vi "CheckPossibleBalls.vi"(1 "max ball vel":dbl, 8 "Fps":dbl=40.0, 9 "Field Size":T3, 10 "Array of cameras":T4[](array[typedef]) {"robots_blue"."height" format="%+4.3f"; "robots_blue"."pixel_y" format="%+4.3f"; "robots_blue"."pixel_x" format="%+4.3f"; "robots_blue"."orientation" format="%+4.3f"; "robots_blue"."y" format="%+4.3f"; "robots_blue"."confidence" format="%4.3f"; "robots_blue"."x" format="%+4.3f"; "robots_yellow"."height" format="%+4.3f"; "robots_yellow"."pixel_y" format="%+4.3f"; "robots_yellow"."pixel_x" format="%+4.3f"; "robots_yellow"."orientation" format="%+4.3f"; "robots_yellow"."y" format="%+4.3f"; "robots_yellow"."confidence" format="%4.3f"; "robots_yellow"."x" format="%+4.3f"}, 11 "last ball choosed by mediacameras":T1[](array[typedef])) -> (2 "sum":i32, 3 "Detection Frame In out":T4[](array[typedef]) {"robots_blue"."height" format="%+4.3f"; "robots_blue"."pixel_y" format="%+4.3f"; "robots_blue"."pixel_x" format="%+4.3f"; "robots_blue"."orientation" format="%+4.3f"; "robots_blue"."y" format="%+4.3f"; "robots_blue"."confidence" format="%4.3f"; "robots_blue"."x" format="%+4.3f"; "robots_yellow"."height" format="%+4.3f"; "robots_yellow"."pixel_y" format="%+4.3f"; "robots_yellow"."pixel_x" format="%+4.3f"; "robots_yellow"."orientation" format="%+4.3f"; "robots_yellow"."y" format="%+4.3f"; "robots_yellow"."confidence" format="%4.3f"; "robots_yellow"."x" format="%+4.3f"})   [LabVIEW 2023]
uses:
  Vision_class/Old vision/Controls/SSL Detection Frame.ctl
  Vision_class/Old vision/Controls/SSL Detection Robot.ctl
  <vilib>/Analysis/Matrix/Datatypes/RealMatrix.ctl
  Vision_class/Old vision/Controls/SSL Detection Ball.ctl
  Utilities_class/Utilities.lvclass
  <vilib>/Analysis/Matrix/NI_Matrix.lvlib
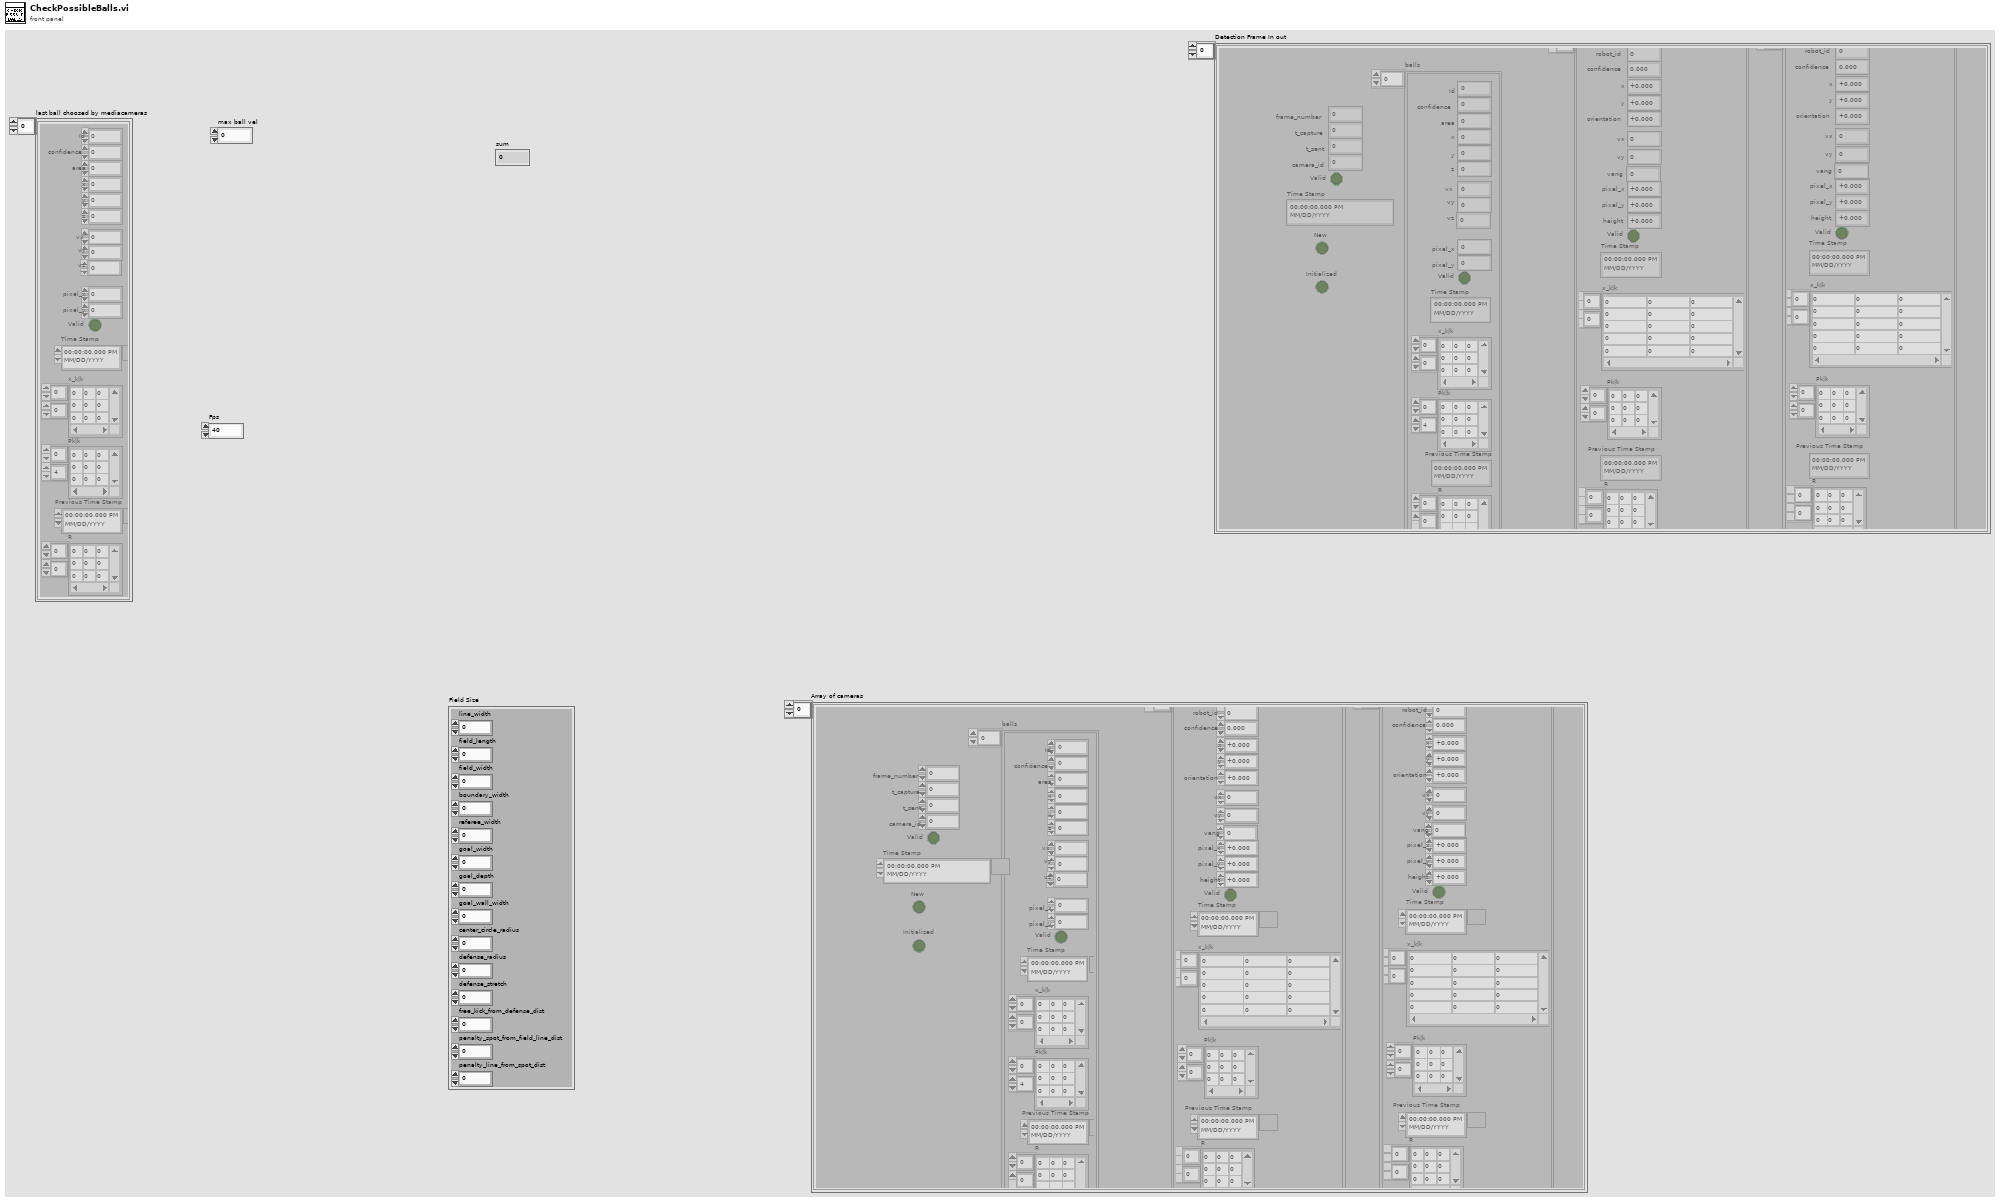
[diagram p1: front panel]
types:
  T1 = typedef "SSL Detection Ball.ctl" = cluster{"x":sgl, "area":u32, "confidence":sgl, "y":sgl, "z":sgl, "pixel_x":sgl, "pixel_y":sgl, "Valid":bool, "Time Stamp":timestamp, "x_k|k":T2, "Pk|k":T2, "Id":u32, "Previous Time Stamp":timestamp, "R":T2, " vx":sgl, "vy":dbl, "vz":dbl}
  T2 = typedef "NI_Matrix.lvlib/RealMatrix.ctl" = dbl[][]
  T3 = cluster{"line_width":u32, "field_length":u32, "field_width":u32, "boundary_width":u32, "referee_width":u32, "goal_width":u32, "goal_depth":u32, "goal_wall_width":u32, "center_circle_radius":u32, "defense_radius":u32, "defense_stretch":u32, "free_kick_from_defense_dist":u32, "penalty_spot_from_field_line_dist":u32, "penalty_line_from_spot_dist":u32}
  T4 = typedef "SSL Detection Frame.ctl" = cluster{"frame_number":u32, "t_capture":dbl, "t_sent":dbl, "camera_id":u32, "robots_yellow":T5[], "robots_blue":T5[], "balls":T1[], "Valid":bool, "Time Stamp":timestamp, "New":bool, "Initialized":bool}
  T5 = typedef "SSL Detection Robot.ctl" = cluster{"x":sgl, "robot_id":u32, "confidence":sgl, "y":sgl, "orientation":sgl, "pixel_x":sgl, "pixel_y":sgl, "height":sgl, "Valid":bool, "Time Stamp":timestamp, "x_k|k":T2, "Pk|k":T2, "Previous Time Stamp":timestamp, "R":T2, "vx":dbl, "vy":dbl, "vang":dbl}
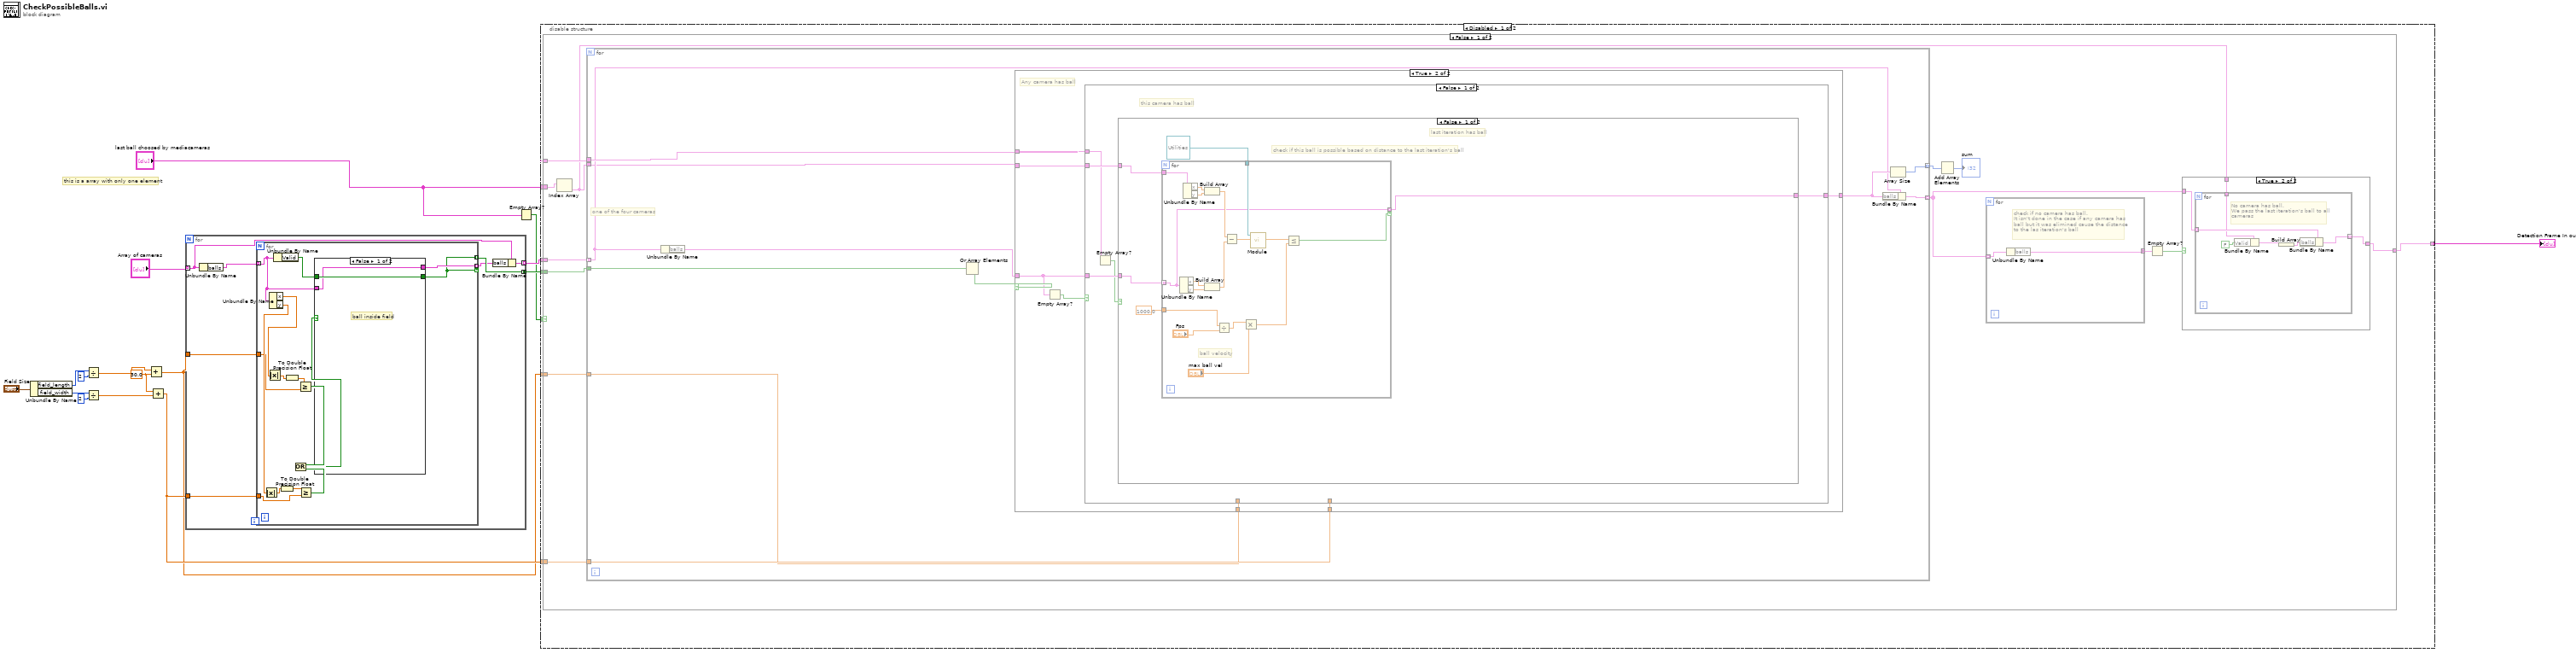
[diagram p0: block diagram]
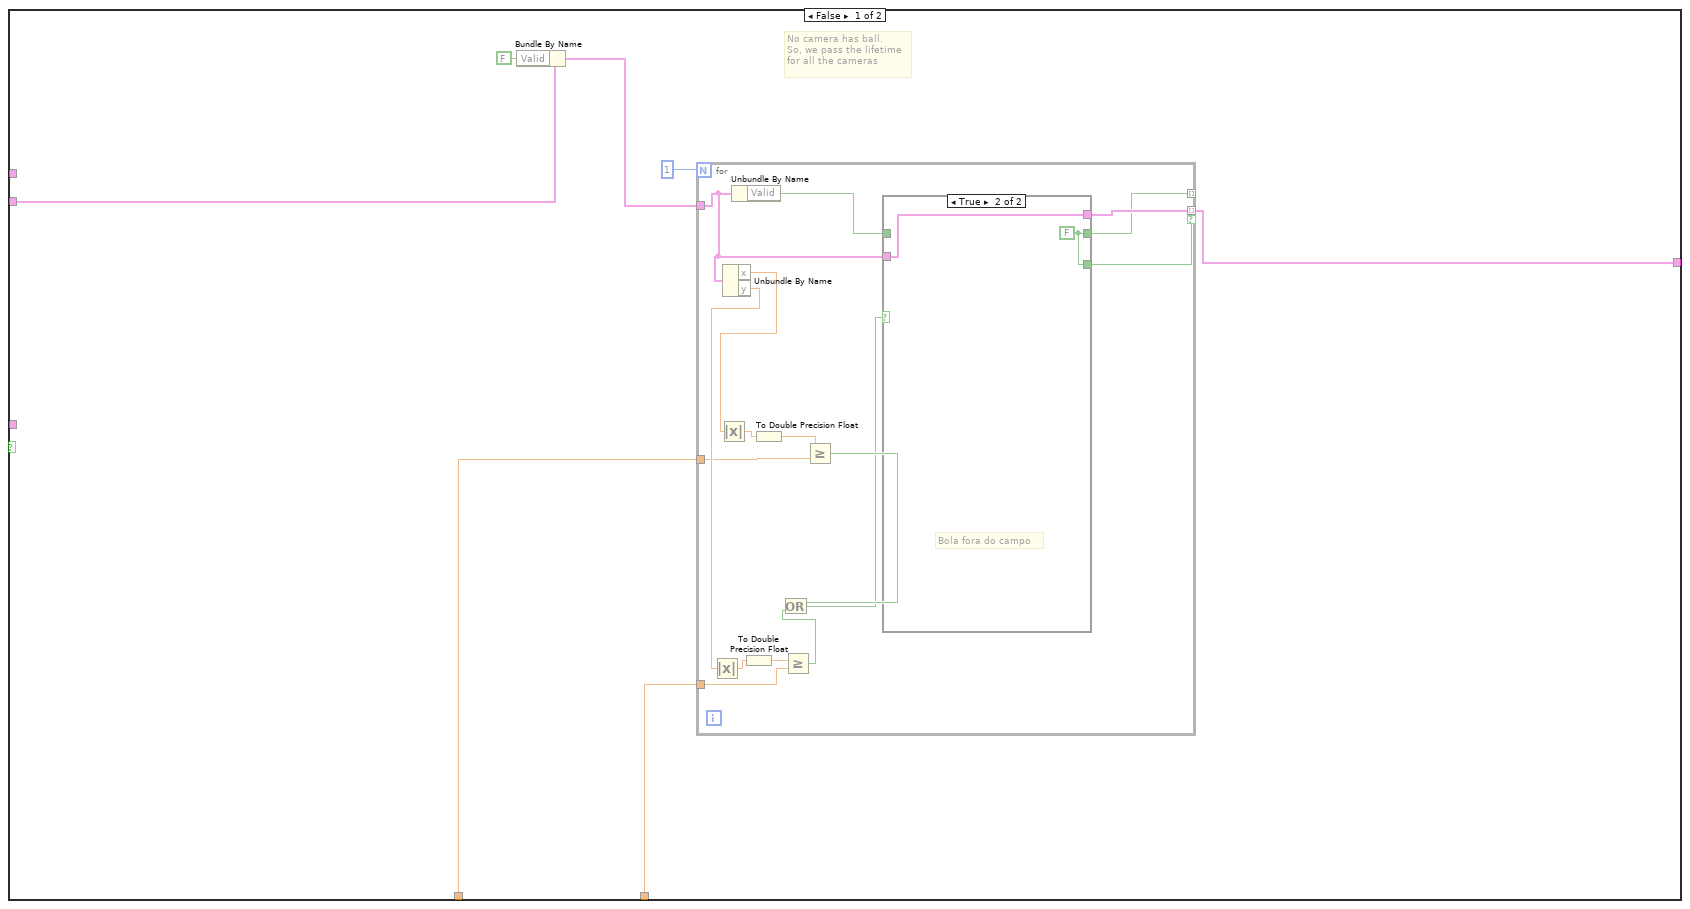
[diagram p3: hidden frame]
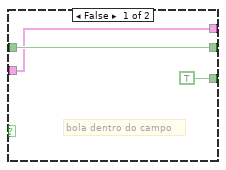
[diagram p4: hidden frame]
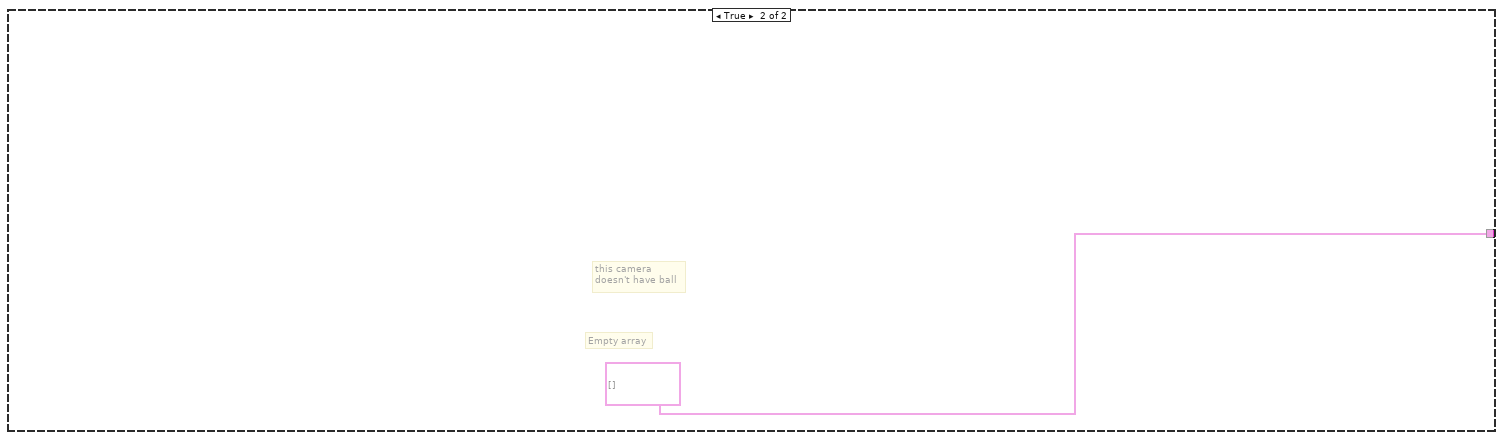
[diagram p6: hidden frame]
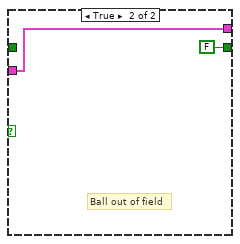
[diagram p9: hidden frame]
diagram:
  w10 = 30.0 ("y")
  # "this is a array with only one element"
  n1 = Unbundle By Name("Field Size") -> ("field_length"=w15:u32, "field_width"=w14:u32)
  n2 = Divide(x=w15, y=2) -> (x/y=w9:dbl)
  n3 = Divide(x=w14, y=2) -> (x/y=w11:dbl)
  n4 = Add(x=w9, y=w10) -> (x+y=w7:dbl)
  n5 = Add(x=w10, y=w11) -> (x+y=w8:dbl)
  n6 = for {
    tunnel: w8 -> [w23]
    tunnel: w7 -> [w22]
    tunnel: "Array of cameras" -> [w18] mode=indexing
    tunnel: [w17] -> w4 mode=indexing
    tunnel: [w20] -> w6 mode=concatenating
    n7 = Unbundle By Name(w18) -> ("balls"=w21:T1[])
    n8 = for {
      tunnel: w21 -> [w29] mode=indexing
      tunnel: [w26] -> w20 mode=indexing
      tunnel: [w37] -> w19 mode=indexing if=w26
      tunnel: w23 -> [w25]
      tunnel: w22 -> [w24]
      n9 = Unbundle By Name(w29) -> ("x"=w28:sgl, "y"=w27:sgl)
      n10 = Absolute Value(x=w27) -> (abs(x)=w33:sgl)
      n11 = Absolute Value(x=w28) -> (abs(x)=w32:sgl)
      n12 = Unbundle By Name(w29) -> ("Valid"=w38:bool)
      n13 = To Double Precision Float(number=w33) -> (double precision float=w34:dbl)
      n14 = To Double Precision Float(number=w32) -> (double precision float=w31:dbl)
      n15 = Greater Or Equal?(x=w31, y=w24) -> (x >= y?=w36:bool)
      n16 = Greater Or Equal?(x=w34, y=w25) -> (x >= y?=w35:bool)
      n17 = Or(x=w36, y=w35) -> (x .or. y?=w30:bool)
      n18 = case shown="False" w30 {
        tunnel: w38 -> [w40 _]
        tunnel: [w40 FALSE ("Valid")] -> w26
        tunnel: w29 -> [w39 w41]
        tunnel: [w39 w41] -> w37
        frame False {
          # "ball inside field"
        }
        frame True {
          # "Ball out of field"
        }
      }
    }
    n19 = Bundle By Name(cluster=w18, "balls"=w19) -> (w17:T4)
  }
  n20 = Empty Array?(array="last ball choosed by mediacameras") -> (empty?=w3:bool)
  n21 = disable-structure shown="Disabled" {
    disable-tunnel: w8 -> [w49 _]
    disable-tunnel: w7 -> [w48 _]
    disable-tunnel: w6 -> [w47 _]
    disable-tunnel: w4 -> [w46 w151]
    disable-tunnel: w3 -> [w45 _]
    disable-tunnel: "last ball choosed by mediacameras" -> [w44 _]
    disable-tunnel: [w43 w151] -> w1
    frame Disabled {
      n22 = case shown="False" w45 {
        tunnel: w49 -> [w60 _]
        tunnel: w48 -> [w59 _]
        tunnel: w47 -> [w58 _]
        tunnel: w44 -> [w54 _]
        tunnel: [w53 w150] -> w43
        tunnel: w46 -> [w52 w150]
        tunnel: w44 -> [w51 _]
        frame False {
          n23 = Index Array(array=w51) -> (element=w50:T1)  [unwired: 1 in]
          n24 = for {
            tunnel: [w84] -> w55 mode=indexing
            tunnel: w54 -> [w83]
            tunnel: [w81] -> w62 mode=indexing
            tunnel: w60 -> [w80]
            tunnel: w59 -> [w79]
            tunnel: w58 -> [w77]
            tunnel: w52 -> [w76] mode=indexing
            tunnel: w50 -> [w75]
            # "one of the four cameras"
            n25 = Unbundle By Name(w76) -> ("balls"=w78:T1[])
            n26 = Or Array Elements(Boolean array=w77) -> (logical OR=w85:bool)
            n27 = case shown="True" w85 {
              tunnel: w78 -> [_ w115]
              tunnel: w75 -> [w92 w120]
              tunnel: w83 -> [_ w118]
              tunnel: [w86 w119] -> w82
              tunnel: w79 -> [w88 w117]
              tunnel: w80 -> [w87 w116]
              frame False {
                # "No camera has ball.\nSo, we pass the lifetime\nfor all the cameras"
                n28 = Bundle By Name(cluster=w92, "Valid"=FALSE) -> (w89:T1)
                n29 = for {
                  N: 1 -> [_]
                  tunnel: w89 -> [w99]
                  tunnel: [w94] -> _ mode=indexing
                  tunnel: [w107] -> w86 mode=indexing if=w93
                  tunnel: w88 -> [w96]
                  tunnel: w87 -> [w95]
                  n30 = Unbundle By Name(w99) -> ("x"=w98:sgl, "y"=w97:sgl)
                  n31 = Absolute Value(x=w97) -> (abs(x)=w103:sgl)
                  n32 = Absolute Value(x=w98) -> (abs(x)=w102:sgl)
                  n33 = Unbundle By Name(w99) -> ("Valid"=w108:bool)
                  n34 = To Double Precision Float(number=w103) -> (double precision float=w104:dbl)
                  n35 = To Double Precision Float(number=w102) -> (double precision float=w101:dbl)
                  n36 = Greater Or Equal?(x=w104, y=w95) -> (x >= y?=w105:bool)
                  n37 = Greater Or Equal?(x=w101, y=w96) -> (x >= y?=w106:bool)
                  n38 = Or(x=w106, y=w105) -> (x .or. y?=w100:bool)
                  n39 = case shown="True" w100 {
                    tunnel: w108 -> [w111 _]
                    tunnel: [w111 w112] -> w94
                    tunnel: w99 -> [w110 w113]
                    tunnel: [w110 w113] -> w107
                    tunnel: [TRUE w112] -> w93
                    frame False {
                      # "bola dentro do campo"
                    }
                    frame True {
                      w112 = FALSE ("Valid")
                      # "Bola fora do campo"
                    }
                  }
                }
              }
              frame True {
                # "Any camera has ball"
                n40 = Empty Array?(array=w115) -> (empty?=w114:bool)
                n41 = case shown="False" w114 {
                  tunnel: w115 -> [w125 _]
                  tunnel: w120 -> [w124 _]
                  tunnel: [w122 T1[] [] ("balls")] -> w119
                  tunnel: w118 -> [w121 _]
                  tunnel: w117 -> [_ _]
                  tunnel: w116 -> [_ _]
                  frame False {
                    # "this camera has ball"
                    n42 = Empty Array?(array=w121) -> (empty?=w123:bool)
                    n43 = case shown="False" w123 {
                      tunnel: w125 -> [w130 w148]
                      tunnel: w124 -> [w129 _]
                      tunnel: [w126 w148] -> w122
                      frame False {
                        # "check if this ball is possible based on distance to the last iteration's ball"
                        # "last iteration has ball"
                        n44 = for {
                          tunnel: w130 -> [w134] mode=indexing
                          tunnel: w129 -> [w147]
                          tunnel: refnum<class "Utilities.lvclass"> refnum ("Utilities in") -> [w140]
                          tunnel: [w134] -> w126 mode=indexing if=w132
                          tunnel: 1000.0 ("x") -> [w133]
                          # "ball velocity"
                          n45 = Unbundle By Name(w134) -> ("x"=w146:sgl, "y"=w145:sgl)
                          n46 = Unbundle By Name(w147) -> ("x"=w144:sgl, "y"=w143:sgl)
                          n47 = Build Array(w144, w143) -> (w142:sgl[])
                          n48 = Build Array(w146, w145) -> (w141:sgl[])
                          n49 = Divide(x=w133, y="Fps") -> (x/y=w136:dbl)
                          n50 = Subtract(x=w142, y=w141) -> (x-y=w139:sgl[])
                          n51 = Multiply(x=w136, y="max ball vel") -> (x*y=w135:dbl)
                          n52 = call-dynamic "Module.vi"("2D vector"=w139, "Utilities in"=w140) -> ("Modulo"=w138:dbl)  [unwired: 7 in, 2 out]
                          n53 = Less Or Equal?(x=w138, y=w135) -> (x <= y?=w132:bool)
                        }
                      }
                      frame True {
                        # "last iteration doesn't have ball,\nincluding the first iteration.\n\nSo, we pass all balls. If it's in this case, that's why this camera has ball."
                      }
                    }
                  }
                  frame True {
                    # "Empty array"
                    # "this camera \ndoesn't have ball"
                  }
                }
              }
            }
            n54 = Bundle By Name(cluster=w76, "balls"=w82) -> (w84:T4)
            n55 = Array Size(array=w82) -> (size(s)=w81:i32)
          }
          n56 = Add Array Elements(numeric array=w62) -> (sum=→"sum":i32)
          n57 = for {
            tunnel: w55 -> [w74] mode=indexing
            tunnel: [w73] -> w57 mode=concatenating
            # "check if no camera has ball.\nIt isn't done in the case if any camera has\nball but it was elimined cause the distance\nto the las iteration's ball"
            n58 = Unbundle By Name(w74) -> ("balls"=w73:T1[])
          }
          n59 = Empty Array?(array=w57) -> (empty?=w56:bool)
          n60 = case shown="True" w56 {
            tunnel: [w63 w65] -> w53
            tunnel: w55 -> [w63 w66]
            tunnel: w50 -> [_ w64]
            frame False {
              # "any camera has ball"
            }
            frame True {
              n61 = for {
                tunnel: w66 -> [w72] mode=indexing
                tunnel: [w71] -> w65 mode=indexing
                tunnel: w64 -> [w69]
                # "No camera has ball.\nWe pass the last iteration's ball to all\ncameras"
                n62 = Bundle By Name(cluster=w69, "Valid"=FALSE) -> (w68:T1)
                n63 = Build Array(w68) -> (w70:T1[])
                n64 = Bundle By Name(cluster=w72, "balls"=w70) -> (w71:T4)
              }
            }
          }
        }
        frame True {
          # "Doesn't have last ball.\n\nPass all inside field"
        }
      }
    }
    frame Enabled {
    }
  }
  "Detection Frame In out" <- w1
